vi "Event Actor.vi"(4 "Queue Nested":map{string, refnum<data-value>}(c390), 6 "Queue Self":map{string, refnum<data-value>}(c390), 8 "Queue Caller":map{string, refnum<data-value>}(c390), 9 "Queue of Event Self":refnum<queue>, 10 "Event Self Alias":string, 11 "Event jettl":refnum<class "Event jettl.lvclass">) -> ()   [LabVIEW 2021, in "jettl.lvlib" / "Base Event jettl.lvlib" / "Base Event jettl.lvclass"]
uses:
  Base Event jettl.lvclass
  Event jettl/Event jettl.lvclass
  Msg Strategy/Msg Strategy.lvclass
  C:/git/jettl/src/jettl/jettl/Event jettl/Event jettl.lvclass
  Event Last Ack/Event Last Ack Msg Strategy/Event Last Ack Msg Strategy.lvclass
  C:/git/jettl/src/jettl/Msg Strategy/Msg Strategy/Msg Strategy.lvclass
  Base Event jettl.lvclass/Base Event jettl.ctl
  jettl.lvlib
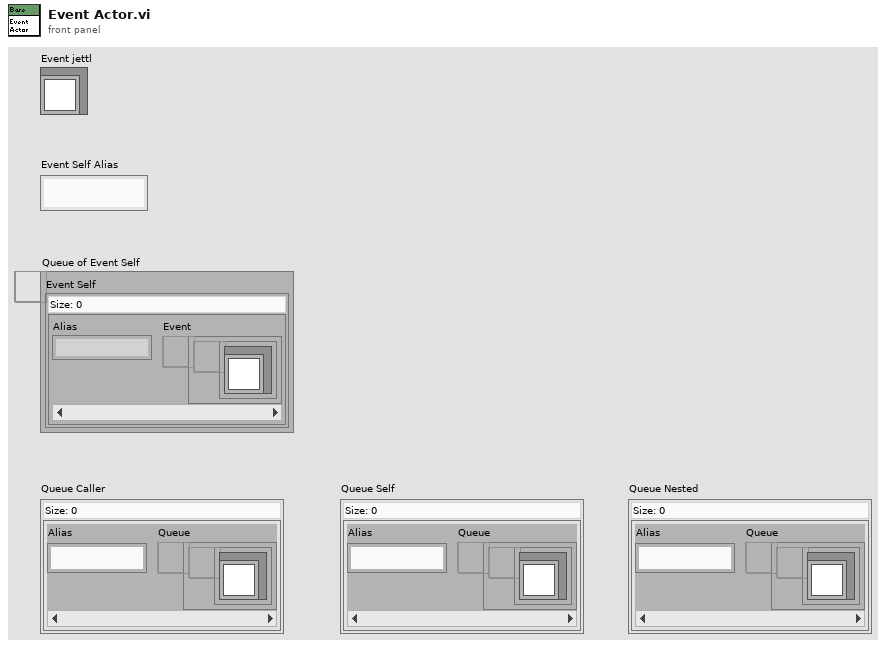
[diagram p1: front panel]
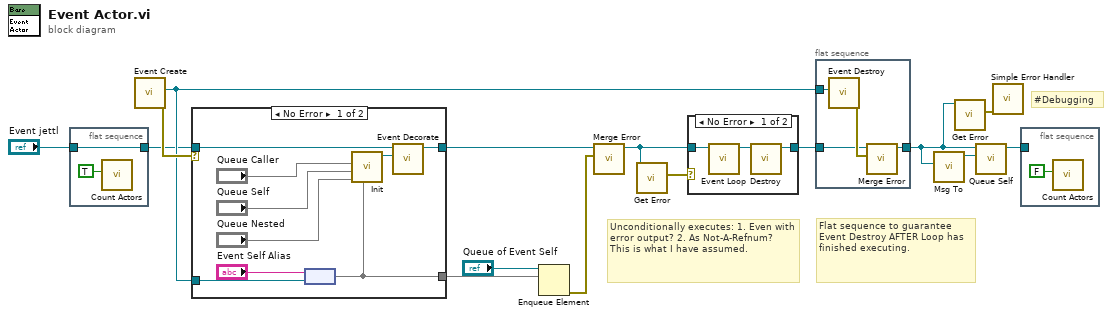
[diagram p0: block diagram]
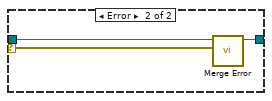
[diagram p2: hidden frame]
diagram:
  # "#Debugging"
  # "Flat sequence to guarantee Event Destroy AFTER Loop has finished executing."
  # "Unconditionally executes: 1. Even with error output? 2. As Not-A-Refnum?\nThis is what I have assumed."
  n1 = flat-sequence {
    tunnel: [w16] -> w2
    tunnel: "Event jettl" -> [w16]
    frame #0 {
      n2 = call "Count Actors.vi"("Increment?"=TRUE) -> ()  [unwired: 11 in]
    }
  }
  n3 = call "Event Create.vi"() -> ("error out"=w9:errorcluster, "Event"=w8:refnum<data-value>)  [unwired: 10 in]
  n4 = case shown="No Error" w9 {
    selector: w9 -> [_ w28]
    tunnel: [w18 w29] -> w13
    tunnel: w2 -> [w25 w27]
    tunnel: w8 -> [w26 _]
    tunnel: [w24 _] -> w12
    frame No Error {
      n5 = node("Event Self Alias", w26) -> (w24:map{string, refnum<data-value>})
      n6 = call "Init.vi"("Event Self"=w24, "Queue Nested"="Queue Nested", "Queue Self"="Queue Self", "Queue Caller"="Queue Caller") -> ("Base Event jettl out"=w19:refnum<class "Base Event jettl.lvclass">)  [unwired: 7 in]
      n7 = call-dynamic "Event Decorate.vi"("Event jettl"=w19, "Event jettl in"=w25) -> ("Event jettl out"=w18:refnum<class "Event jettl.lvclass">)  [unwired: 9 in]
    }
    frame Error {
      n8 = call-dynamic "Merge Error.vi"("Error"=w28, "Merge Error in"=w27) -> ("Merge Error out"=w29:refnum<class "Event jettl.lvclass">)  [unwired: 9 in]
    }
  }
  n9 = Enqueue Element(queue="Queue of Event Self", element=w12) -> (error out=w14:errorcluster)  [unwired: 2 in, 2 out]
  n10 = call-dynamic "Merge Error.vi"("Error"=w14, "Merge Error in"=w13) -> ("Merge Error out"=w15:refnum<class "Event jettl.lvclass">)  [unwired: 9 in]
  n11 = call-dynamic "Get Error.vi"("jettl in"=w15) -> ("Error"=w11:errorcluster)  [unwired: 10 in]
  n12 = case shown="No Error" w11 {
    tunnel: w15 -> [w30 w33]
    tunnel: [w32 w33] -> w10
    frame No Error {
      n13 = call-dynamic "Event Loop.vi"("Event jettl in"=w30) -> ("Event jettl out"=w31:refnum<class "Event jettl.lvclass">)  [unwired: 10 in]
      n14 = call-dynamic "Destroy.vi"("jettl in"=w31) -> ("jettl out"=w32:refnum<class "Event jettl.lvclass">)  [unwired: 10 in]
    }
    frame Error {
    }
  }
  n15 = flat-sequence {
    tunnel: w8 -> [w36]
    tunnel: [w37] -> w4
    tunnel: w10 -> [w34]
    frame #0 {
      n16 = call "Event Destroy.vi"("Event"=w36) -> ("error out"=w35:errorcluster)  [unwired: 10 in]
      n17 = call-dynamic "Merge Error.vi"("Error"=w35, "Merge Error in"=w34) -> ("Merge Error out"=w37:refnum<class "Event jettl.lvclass">)  [unwired: 9 in]
    }
  }
  n18 = call "Msg To.vi"("Event jettl"=w4) -> ("Event Last Ack Msg Strategy out"=w6:refnum<class "Event Last Ack Msg Strategy.lvclass">)  [unwired: 10 in]
  n19 = call-dynamic "Get Error.vi"("jettl in"=w4) -> ("Error"=w5:errorcluster)  [unwired: 10 in]
  n20 = call-dynamic "Queue Self.vi"("Msg Strategy"=w6, "jettl in"=w4) -> ("jettl out"=w1:refnum<class "Event jettl.lvclass">)  [unwired: 9 in]
  n21 = call <vilib>:"Simple Error Handler.vi"("error in (no error)"=w5) -> ()  [unwired: 4 in, 5 out]
  n22 = flat-sequence {
    tunnel: w1 -> [_]
    frame #0 {
      n23 = call "Count Actors.vi"("Increment?"=FALSE) -> ()  [unwired: 11 in]
    }
  }
